vi "PXI-2510.Async.vi"(10 "Parameters":variant, 11 "Process":refnum<class "Process.lvclass">) -> ()   [LabVIEW 2020, in "PXI-2510 Engine.lvlib"]
uses:
  PXI-2510 Engine.lvlib
  <vilib>/NI/NIVS Inline Async API/_VS Inline Async API/Process/Process.lvclass
  <instrlib>/niSwitch/niSwitch.llb/niSwitch Topologies.ctl
  Shared/Compiled.Settings.ctl
  <vilib>/NI/NIVS Inline Async API/_VS Inline Async API/Process/Process.lvclass/Process.ctl
  <vilib>/NI/NIVS Inline Async API/_Data Access Engine/Access Type Classes/Read/Read.lvclass/Read.ctl
  <vilib>/NI/NIVS Inline Async API/_Data Access Engine/Access Type Classes/Write/Write.lvclass/Write.ctl
  <vilib>/NI/NIVS Inline Async API/_Data Access Engine/Data Access Engine/Methods/Read.Data.vi
  <vilib>/NI/NIVS Inline Async API/_VS Inline Async API/Process/Data Member Access/Read Data Access.vi
  <vilib>/NI/NIVS Inline Async API/_VS Inline Async API/Error Handling Process/SubVIs/Error.ConvertArray.vi
  <vilib>/NI/NIVS Inline Async API/_Data Access Engine/Access Type Classes/Read/Read.ProcessData.vi
  <vilib>/NI/NIVS Inline Async API/_Data Access Engine/Access Type Classes/Write/Write.ProcessData.vi
  <vilib>/NI/NIVS Inline Async API/_Data Access Engine/Access Type Classes/Write/Write.Buffer.vi
  <vilib>/NI/NIVS Inline Async API/_Data Access Engine/Access Type Classes/Write/Write.Commit.vi
  <vilib>/NI/NIVS Inline Async API/_Data Access Engine/Data Access Engine/Methods/Read.Lookup.vi
  <vilib>/NI/NIVS Inline Async API/_Data Access Engine/Data Access Engine/Methods/Write.Lookup.vi
  <vilib>/NI/NIVS Inline Async API/_Data Access Engine/Data Access Engine/Data Access Engine.lvclass
  Shared/PXI-2510 Shared.lvlib
  <vilib>/NI/NIVS Inline Async API/_Data Access Engine/Data Access Engine/Methods/Write.Data.vi
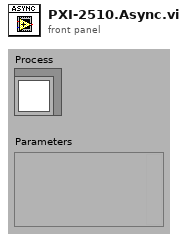
[diagram p1: front panel]
types:
  T1 = typedef "niSwitch Topologies.ctl" = string
  T2 = typedef "PXI-2510 Shared.lvlib/Compiled.Settings.ctl" = cluster{"Name":string, "Async Init Timeout":u16, "Hardware Device Name":string}
  T3 = typedef "Data Access Engine.lvlib/Data Access Engine.lvclass/Read.DVR.ctl" = refnum<data-value>
  T4 = typedef "Data Access Engine.lvlib/Data Access Engine.lvclass/Write.DVR.ctl" = refnum<data-value>
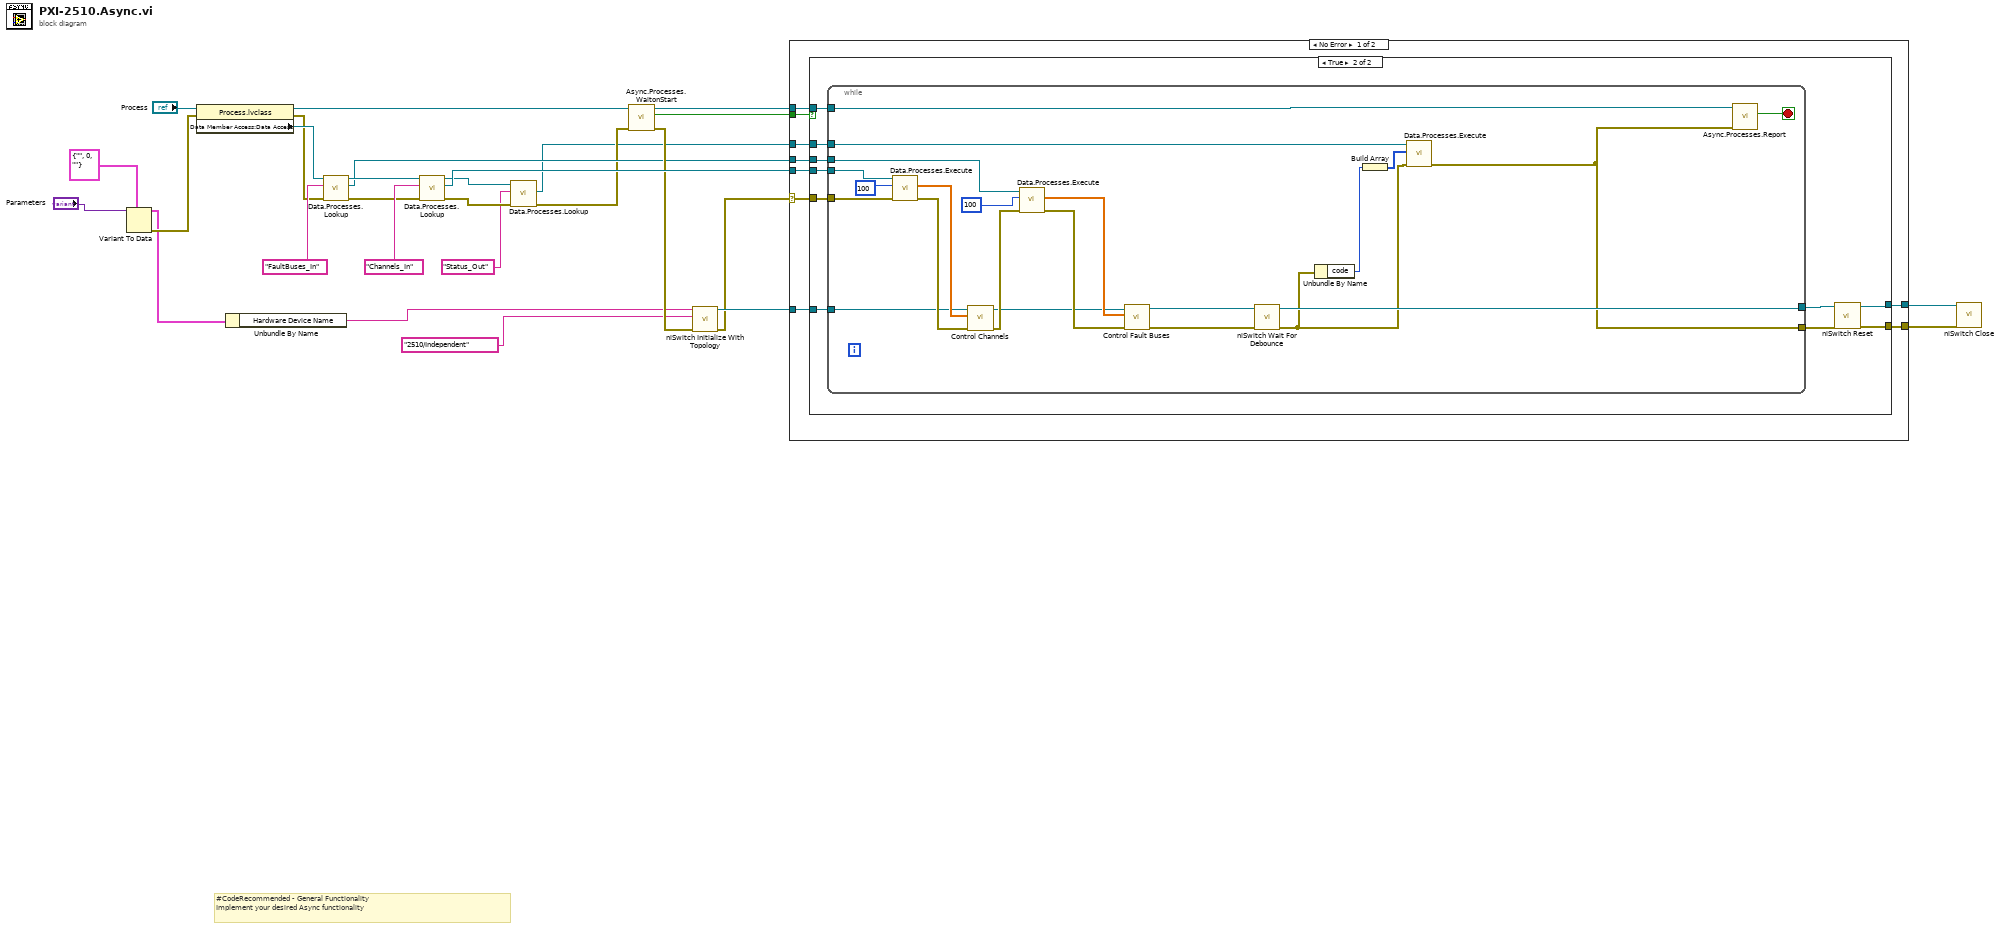
[diagram p0: block diagram]
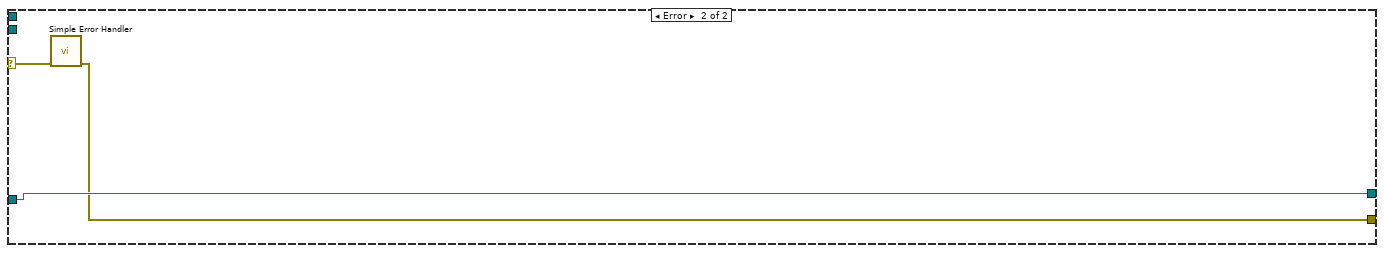
[diagram p3: hidden frame]
diagram:
  # "#CodeRecommended - General Functionality\nImplement your desired Async functionality"
  n1 = Variant To Data(type=T2 {"Name"="", "Async Init Timeout"=0, "Hardware Device Name"=""} ("Compiled.Settings"), Variant="Parameters") -> (data=w13:T2, error out=w15:errorcluster)  [unwired: 1 in]
  n2 = property class="Process.lvclass"(reference="Process", error in=w15) -> (reference out=w20:refnum<class "Process.lvclass">, error out=w18:errorcluster, "Data Member Access:Data Access"=w19:refnum<class "Data Access Engine.lvclass">)
  n3 = Unbundle By Name(w13) -> ("Hardware Device Name"=w12:string)
  n4 = call-poly <vilib>:"Data.Processes.Lookup.vi"("error in (no error)"=w18, "Name"="FaultBuses_In", "Data Access API in"=w19) -> ("error out"=w23:errorcluster, "Ref"=w8:T3, "Data Access API out"=w22:refnum<class "Data Access Engine.lvclass">)  [unwired: 5 in, 1 out]
  n5 = call-poly <vilib>:"Data.Processes.Lookup.vi"("error in (no error)"=w23, "Name"="Channels_In", "Data Access API in"=w22) -> ("error out"=w5:errorcluster, "Ref"=w25:T3, "Data Access API out"=w4:refnum<class "Data Access Engine.lvclass">)  [unwired: 5 in, 1 out]
  n6 = call-poly <vilib>:"Data.Processes.Lookup.vi"("error in (no error)"=w5, "Name"="Status_Out", "Data Access API in"=w4) -> ("error out"=w3:errorcluster, "Ref"=w2:T4)  [unwired: 5 in, 2 out]
  n7 = call <vilib>:"Async.Processes.WaitonStart.vi"("error in (no error)"=w3, "Process"=w20) -> ("error out"=w14:errorcluster, "Execute"=w28:bool, "Process out"=w27:refnum<class "Process.lvclass">)  [unwired: 7 in]
  n8 = call <instrlib>:"niSwitch Initialize With Topology.vi"("error in (no error)"=w14, "topology name"=T1 "2510/Independent", "resource name"=w12) -> ("error out"=w9:errorcluster, "instrument handle out"=w10:refnum<k15>)  [unwired: 7 in]
  n9 = case shown="No Error" w9 {
    selector: w9 -> [w34 w74]
    tunnel: w28 -> [w37 _]
    tunnel: w27 -> [w36 _]
    tunnel: w25 -> [w35 _]
    tunnel: w10 -> [w33 w73]
    tunnel: [w32 w73] -> w7
    tunnel: w8 -> [w31 _]
    tunnel: [w30 w72] -> w6
    tunnel: w2 -> [w29 _]
    frame No Error {
      n10 = case shown="True" w37 {
        tunnel: w34 -> [w38 w47]
        tunnel: w36 -> [_ w48]
        tunnel: w35 -> [_ w49]
        tunnel: w33 -> [w39 w46]
        tunnel: [w39 w45] -> w32
        tunnel: w31 -> [_ w42]
        tunnel: [w38 w41] -> w30
        tunnel: w29 -> [_ w40]
        frame False {
        }
        frame True {
          n11 = while {
            tunnel: w47 -> [w64]
            tunnel: w48 -> [w71]
            tunnel: w49 -> [w69]
            tunnel: w46 -> [w62]
            tunnel: [w55] -> w44
            tunnel: [w52] -> w43
            tunnel: w42 -> [w59]
            tunnel: w40 -> [w54]
            stop <- w70 stop-if-true
            n12 = call-poly <vilib>:"Data.Processes.Execute.vi"("error in (no error)"=w64, "timeout ms"=100, "Ref"=w69) -> ("error out"=w66:errorcluster, "Values"=w67:dbl[])  [unwired: 6 in, 1 out]
            n13 = call "Control Channels.vi"("error in (no error)"=w66, "Values"=w67, "IVI Refnum in"=w62) -> ("error out"=w61:errorcluster, "IVI Refnum out"=w58:refnum<k15>)  [unwired: 7 in]
            n14 = call-poly <vilib>:"Data.Processes.Execute.vi"("error in (no error)"=w61, "timeout ms"=100, "Ref"=w59) -> ("error out"=w60:errorcluster, "Values"=w63:dbl[])  [unwired: 6 in, 1 out]
            n15 = call "Control Fault Buses.vi"("error in (no error)"=w60, "Values"=w63, "IVI Refnum in"=w58) -> ("error out"=w57:errorcluster, "IVI Refnum out"=w56:refnum<k15>)  [unwired: 7 in]
            n16 = call <instrlib>:"niSwitch Wait For Debounce.vi"("error in (no error)"=w57, "instrument handle"=w56) -> ("error out"=w53:errorcluster, "instrument handle out"=w55:refnum<k15>)  [unwired: 8 in]
            n17 = Unbundle By Name(w53) -> ("code"=w50:i32)
            n18 = Build Array(w50) -> (w51:i32[])
            n19 = call-poly <vilib>:"Data.Processes.Execute.vi"("error in (no error)"=w53, "Values"=w51, "Ref"=w54) -> ("error out"=w52:errorcluster)  [unwired: 8 in]
            n20 = call <vilib>:"Async.Processes.Report.vi"("Error"=w52, "Process in"=w71) -> ("Stop"=w70:bool)  [unwired: 8 in, 1 out]
          }
          n21 = call <instrlib>:"niSwitch Reset.vi"("error in (no error)"=w43, "instrument handle"=w44) -> ("error out"=w41:errorcluster, "instrument handle out"=w45:refnum<k15>)  [unwired: 8 in]
        }
      }
    }
    frame Error {
      n22 = call <vilib>:"Simple Error Handler.vi"("error in (no error)"=w74) -> ("error out"=w72:errorcluster)  [unwired: 4 in, 4 out]
    }
  }
  n23 = call <instrlib>:"niSwitch Close.vi"("error in (no error)"=w6, "instrument handle"=w7) -> ()  [unwired: 9 in, 1 out]
